vi "Write pubSubDataEvent.vi"(10 "pubSubDataEvent in":refnum<class "PubSubDataEvent.lvclass">, 11 "MiddlewareSALThisComponent.lvclass in":refnum<class "MiddlewareSALThisComponent.lvclass">) -> (3 "MiddlewareSALThisComponent.lvclass out":refnum<class "MiddlewareSALThisComponent.lvclass">)   [LabVIEW 2016, in "MiddlewareSALThisComponent.lvclass"]
uses:
  MiddlewareSALThisComponent.lvclass
  PubSubDataEvent/PubSubDataEvent.lvclass
  MiddlewareSALThisComponent.lvclass/MiddlewareSALThisComponent.ctl
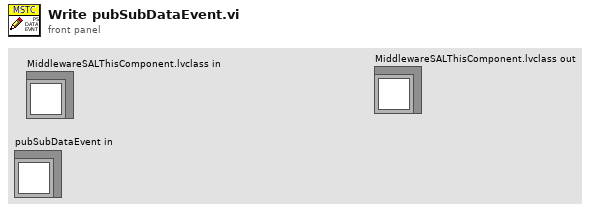
[diagram p1: front panel]
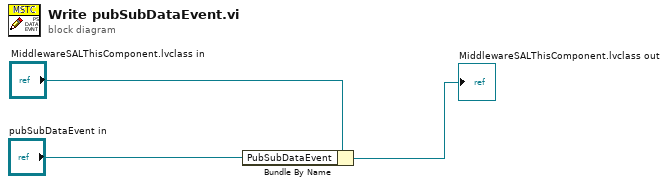
[diagram p0: block diagram]
diagram:
  n1 = Bundle By Name(cluster="MiddlewareSALThisComponent.lvclass in", "PubSubDataEvent"="pubSubDataEvent in") -> (→"MiddlewareSALThisComponent.lvclass out":refnum<class "MiddlewareSALThisComponent.lvclass">)
